vi "Download and Install Shared Binaries.vi"   [LabVIEW 2020]
uses:
  binary_installation_tools/binary_installation_tools.lvlib
  common/common.lvlib
types:
  T1 = typedef "binary_installation_tools.lvlib/Binary Dependency Platform.ctl" = enum16{"Windows Desktop x86", "Windows Desktop x64", "Linux Desktop x64", "Linux Desktop armv8a-rpi5", "NI Linux RT x64", "NI Linux RT armv7a"}
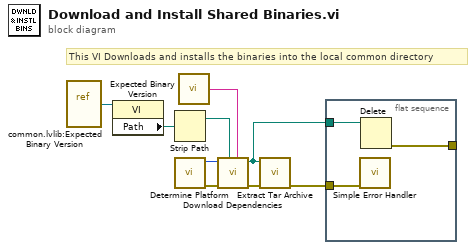
[diagram p0: block diagram]
diagram:
  # "This VI Downloads and installs the binaries into the local common directory"
  n1 = vi-ref "common.lvlib:Expected Binary Version.vi"() -> (w5:refnum<vi>)
  n2 = property class="VI"(reference=w5) -> ("Path"=w4:path)  [unwired: 1 in, 2 out]
  n3 = Strip Path(path=w4) -> (stripped path=w3:path)  [unwired: 1 out]
  n4 = call "Determine Platform.vi"() -> ("error out"=w9:errorcluster, "Platform"=w8:T1)  [unwired: 10 in]
  n5 = call "Expected Binary Version.vi"() -> ("Expected Version"=w2:string)
  n6 = call "Download Dependencies.vi"("Version"=w2, "Target Directory"=w3, "error in (no error)"=w9, "Platform"=w8) -> ("error out"=w7:errorcluster, "Downloaded File"=w1:path)  [unwired: 6 in]
  n7 = call "Extract Tar Archive.vi"("error in (no error)"=w7, "File"=w1) -> ("error out"=w6:errorcluster)  [unwired: 8 in, 1 out]
  n8 = flat-sequence {
    tunnel: w6 -> [w12]
    tunnel: w1 -> [w11]
    tunnel: [w10] -> _
    frame #0 {
      n9 = call <vilib>:"Simple Error Handler.vi"("error in (no error)"=w12) -> ()  [unwired: 4 in, 5 out]
      n10 = Delete(path (use dialog)=w11) -> (error out=w10:errorcluster)  [unwired: 4 in, 2 out]
    }
  }
